vi "CSM Execute - Highlight All Scripts.vi"(6 "Mouse Position":T1, 8 "User VI Ref":refnum<vi>, 9 "Menu Item Tag Suffix":string, 10 "Remaining Items":refnum<vi>[](array[refnum]), 11 "Affected Items":T2) -> (0 "Fail transaction?":bool)   [LabVIEW 2017]
doc: "This VI is part of a plug-in for modifying the LabVIEW shortcut menus. This is the execute VI which is called when the shortcut menu is chosen by the user. It performs the action of the selected menu item."
uses:
  CSM Execute - Shortcut Menu Plug-In.ctl
  <vilib>/Utility/miscctls.llb/LVPositionTypeDef.ctl
  <vilib>/Utility/traverseref.llb/TRef TravTarget.ctl
  <vilib>/Utility/traverseref.llb/VI Scripting - Traverse.lvlib
panel:
  # "All controls on this panel except \"Affected Items\" have been locked to prevent accidental edits. Changing the control names or types, other than the elements of the \"Affected Items\" cluster will make the VI unusable as a menu plugin.\n\nSee Context Help for each control for details about its use."
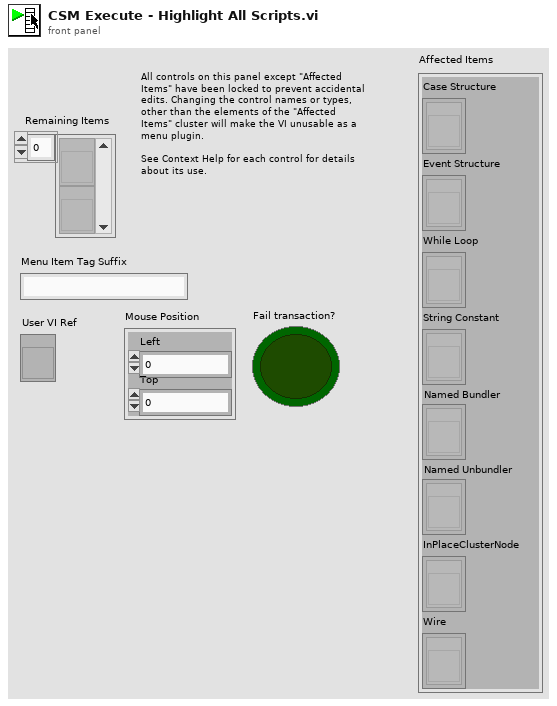
[diagram p1: front panel]
types:
  T1 = typedef "LVPositionTypeDef.ctl" = cluster{"Left":i32, "Top":i32}
  T2 = typedef "CSM Execute - Shortcut Menu Plug-In.ctl" = cluster{"Case Structure":refnum<vi>[], "Event Structure":refnum<vi>[], "While Loop":refnum<vi>[], "String Constant":refnum<vi>[], "Named Bundler":refnum<vi>[], "Named Unbundler":refnum<vi>[], "InPlaceClusterNode":refnum<vi>[], "Wire":refnum<vi>[]}
  T3 = typedef "TRef TravTarget.ctl" = enum16{"FP", "BD", "Other"}
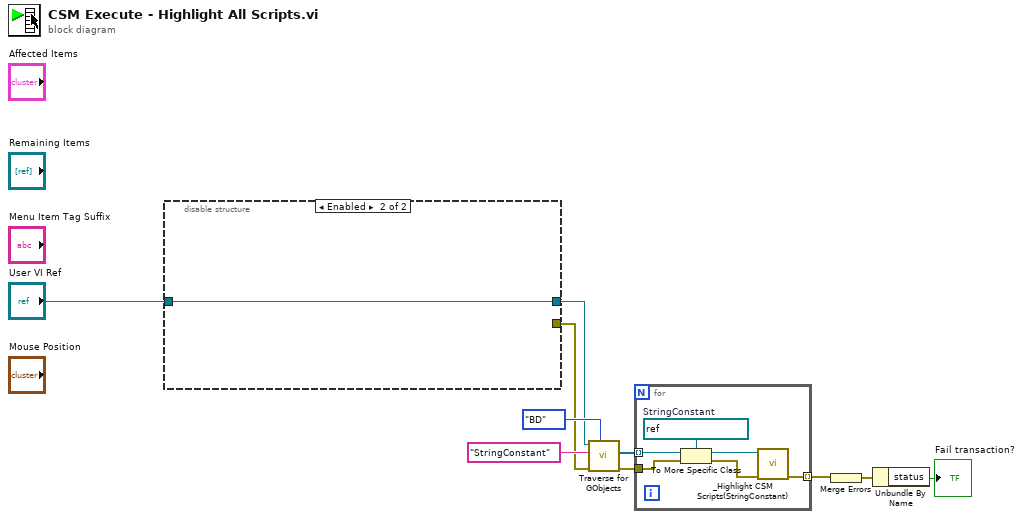
[diagram p0: block diagram]
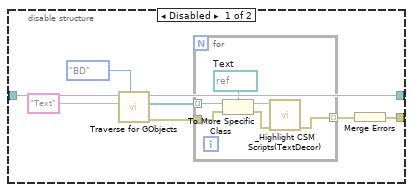
[diagram p2: hidden frame]
diagram:
  n1 = disable-structure shown="Enabled" {
    disable-tunnel: "User VI Ref" -> [w14 w25]
    disable-tunnel: [w13 w25] -> w5
    disable-tunnel: [w11 _] -> w2
    frame Disabled {
      n2 = call <vilib>:"Traverse for GObjects.vi"("Traverse Target"=TRef_TravTarget."BD", "Class Name"="Text", "VI Refnum"=w14) -> ("error out"=w12:errorcluster, "References"=w16:refnum<vi>[], "dup VI Refnum"=w13:refnum<vi>)  [unwired: 5 in, 1 out]
      n3 = for {
        tunnel: w16 -> [w21] mode=indexing
        tunnel: w12 -> [w20]
        tunnel: [w19] -> w15 mode=indexing
        w24 = refnum<vi> refnum  # Text
        n4 = To More Specific Class(target class=w24, reference=w21, error in=w20) -> (specific class reference=w23:refnum<vi>, error out=w22:errorcluster)
        n5 = call "_Highlight CSM Scripts(TextDecor).vi"("error in (no error)"=w22, "Reference Out 2"=w23) -> ("error out"=w19:errorcluster)  [unwired: 9 in]
      }
      n6 = Merge Errors(w15) -> (w11:errorcluster)
    }
    frame Enabled {
    }
  }
  n7 = call <vilib>:"Traverse for GObjects.vi"("Traverse Target"=TRef_TravTarget."BD", "error in (no error)"=w2, "Class Name"="StringConstant", "VI Refnum"=w5) -> ("error out"=w1:errorcluster, "References"=w9:refnum<vi>[])  [unwired: 4 in, 2 out]
  n8 = for {
    tunnel: w9 -> [w31] mode=indexing
    tunnel: w1 -> [w30]
    tunnel: [w26] -> w4 mode=indexing
    w29 = refnum<vi> refnum  # StringConstant
    n9 = To More Specific Class(target class=w29, reference=w31, error in=w30) -> (specific class reference=w28:refnum<vi>, error out=w27:errorcluster)
    n10 = call "_Highlight CSM Scripts(StringConstant).vi"("error in (no error)"=w27, "Reference Out"=w28) -> ("error out"=w26:errorcluster)  [unwired: 9 in]
  }
  n11 = Merge Errors(w4) -> (w3:errorcluster)
  n12 = Unbundle By Name(w3) -> ("status"=→"Fail transaction?":bool)
